vi "Timing Palette.vi"   [LabVIEW 2017]
uses:
  6d46d3cc-b997-40b5-b1a7-ea3ee7b37ab1.vi
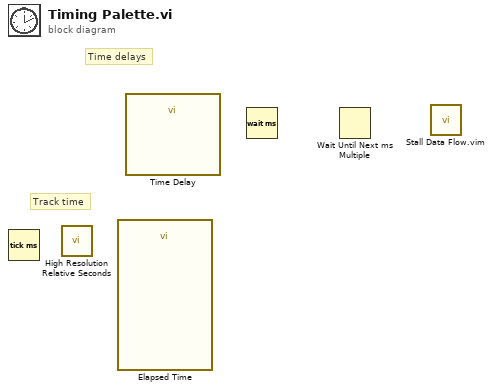
[diagram p0: block diagram]
diagram:
  # "Track time"
  # "Time delays"
  n1 = Tick Count (ms)() -> ()  [unwired: 1 out]
  n2 = call <vilib>:"High Resolution Relative Seconds.vi"() -> ()  [unwired: 1 out]
  n3 = call "Elapsed Time"() -> ()  [unwired: 12 in, 8 out]
  n4 = call "Time Delay"() -> ()  [unwired: 11 in, 1 out]
  n5 = Wait (ms)() -> ()  [unwired: 1 in, 1 out]
  n6 = Wait Until Next ms Multiple() -> ()  [unwired: 1 in, 1 out]
  n7 = call "Stall Data Flow.vim"() -> ()  [unwired: 2 in, 2 out]
